vi "Up and Down POV.vi"(10 "POV":i16) -> (1 "Go Down?":bool, 2 "Go Up?":bool)   [LabVIEW 2014]
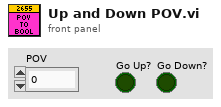
[diagram p1: front panel]
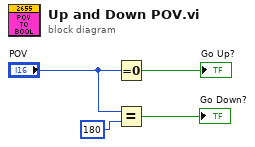
[diagram p0: block diagram]
diagram:
  n1 = Equal To 0?(x="POV") -> (x = 0?=→"Go Up?":bool)
  n2 = Equal?(x="POV", y=i16 180) -> (x = y?=→"Go Down?":bool)
